vi "handler_file.vi"(8 "error in (no error)":errorcluster, 10 "Server Variables":T1 {"Energy Levels"."E1" format="%_6g"; "Phases"."ExtTriggerDelay" format="%.3g"}, 11 "HTTP Request":T7) -> (0 "error out":errorcluster, 2 "Server Variables 2":T1 {"Energy Levels"."E1" format="%_6g"; "Phases"."ExtTriggerDelay" format="%.3g"}, 3 "HTTP Request out":T7)   [LabVIEW 2011]
uses:
  http_request_response.ctl
  http_request.ctl
  http_field.ctl
  http_response.ctl
  template_field.ctl
  template_field_type.ctl
  Server Variables.ctl
  Phase Parameters.ctl
  Phase Mode.ctl
  Energy Level_.ctl
  Measurement Parameters.ctl
  Results.ctl
  <vilib>/regexp/Match Regular Expression.xnode
panel:
  in  "base path":path=path "c:/nanolyzer/www"
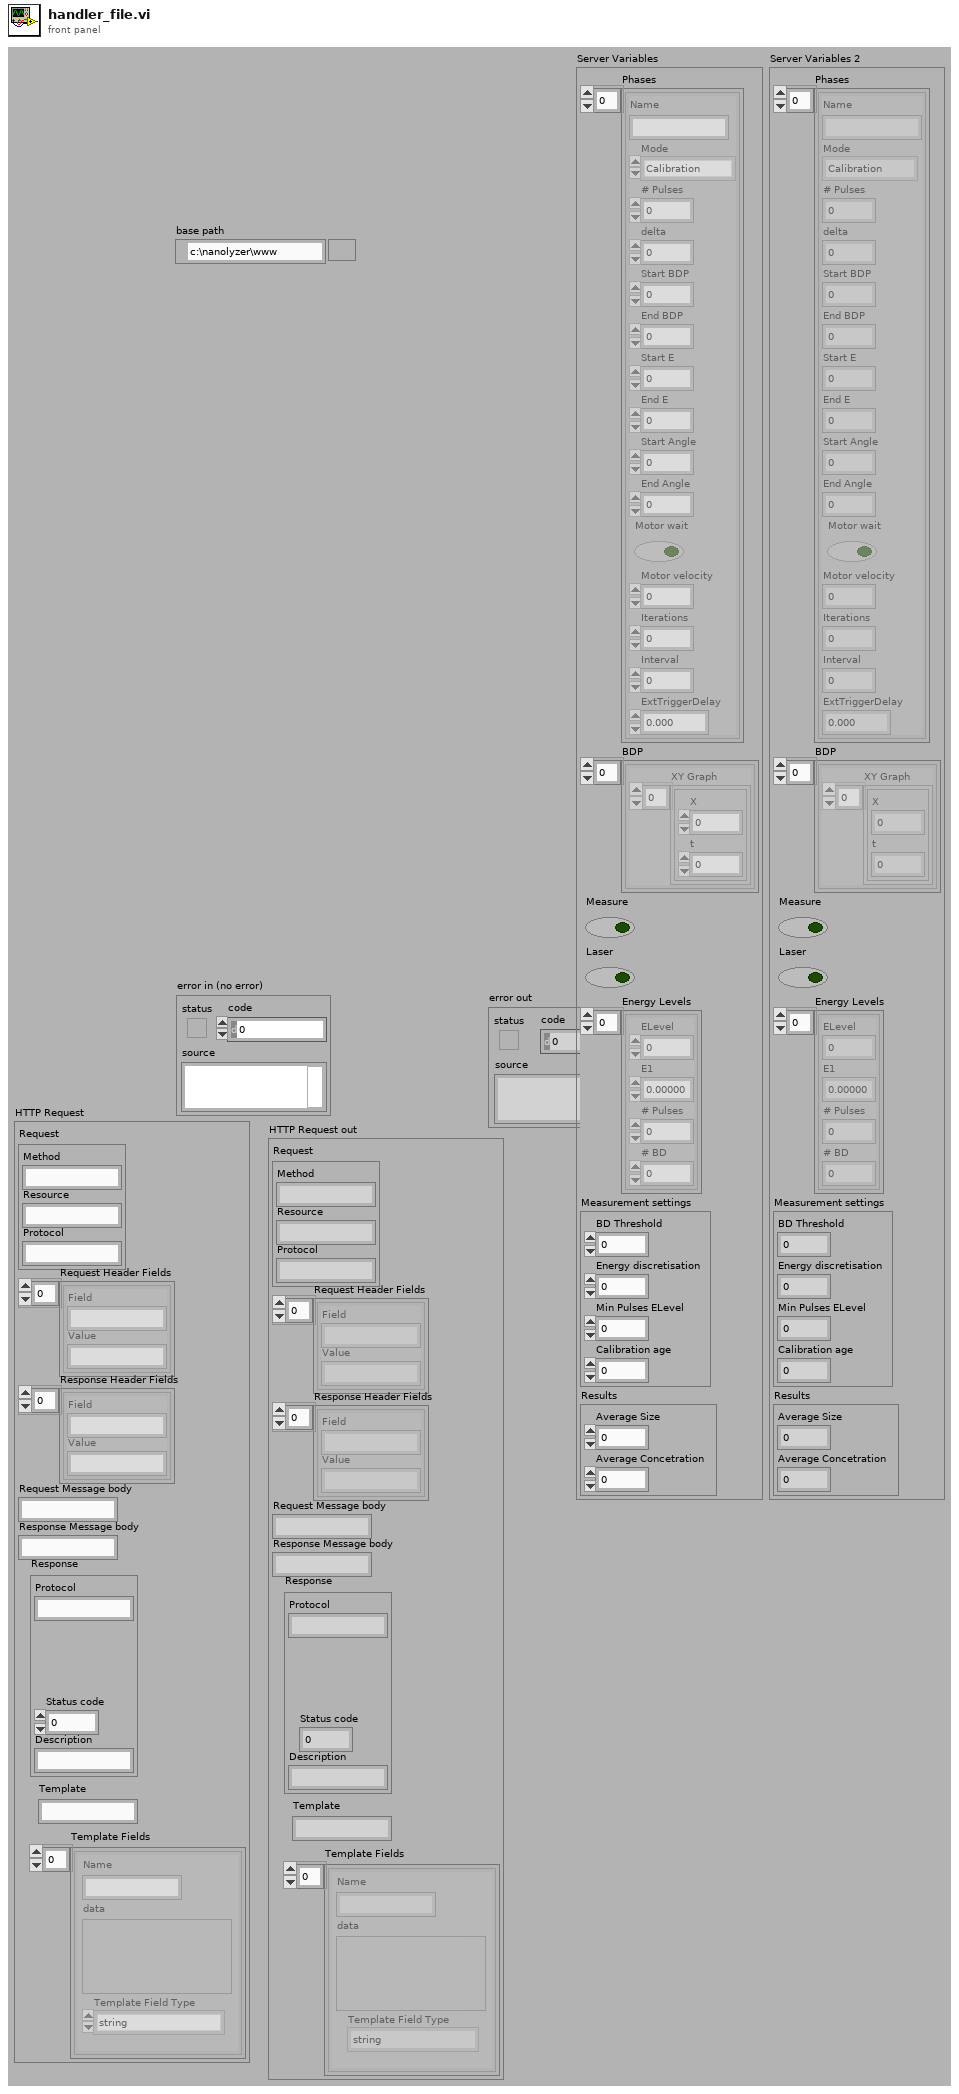
[diagram p1: front panel]
types:
  T1 = typedef "Server Variables.ctl" = cluster{"Phases":T2[], "BDP":cluster{"XY Graph":cluster{"X":dbl, "t":dbl}[]}[], "Measure":bool, "Laser":bool, "Energy Levels":T4[], "Measurement settings":T5, "Results":T6}
  T2 = typedef "Phase Parameters.ctl" = cluster{"Name":string, "Mode":T3, "# Pulses":u32, "delta":dbl, "Start BDP":dbl, "End BDP":dbl, "Start E":dbl, "End E":dbl, "Start Angle":dbl, "End Angle":dbl, "Motor wait":bool, "Motor velocity":dbl, "Iterations":dbl, "Interval":dbl, "ExtTriggerDelay":dbl}
  T3 = typedef "Phase Mode.ctl" = enum16{"Calibration", "Linear", "BDP-Fit", "Raw"}
  T4 = typedef "Energy Level_.ctl" = cluster{"ELevel":dbl, "E1":dbl, "# Pulses":i32, "# BD":i32}
  T5 = typedef "Measurement Parameters.ctl" = cluster{"BD Threshold":dbl, "Energy discretisation":i32, "Min Pulses ELevel":i32, "Calibration age":i32}
  T6 = typedef "Results.ctl" = cluster{"Average Size":dbl, "Average Concetration":dbl}
  T7 = typedef "http_request_response.ctl" = cluster{"Request":T8, "Request Header Fields":T9[], "Response Header Fields":T9[], "Request Message body":string, "Response Message body":string, "Response":T10, "Template":string, "Template Fields":T11[]}
  T8 = typedef "http_request.ctl" = cluster{"Method":string, "Resource":string, "Protocol":string}
  T9 = typedef "http_field.ctl" = cluster{"Field":string, "Value":string}
  T10 = typedef "http_response.ctl" = cluster{"Protocol":string, "Status code":dbl, "Description":string}
  T11 = typedef "template_field.ctl" = cluster{"Name":string, "Template Field Type":T12, "data":variant}
  T12 = typedef "template_field_type.ctl" = enum16{"string", "string array", "number", "number array", "cluster", "cluster array"}
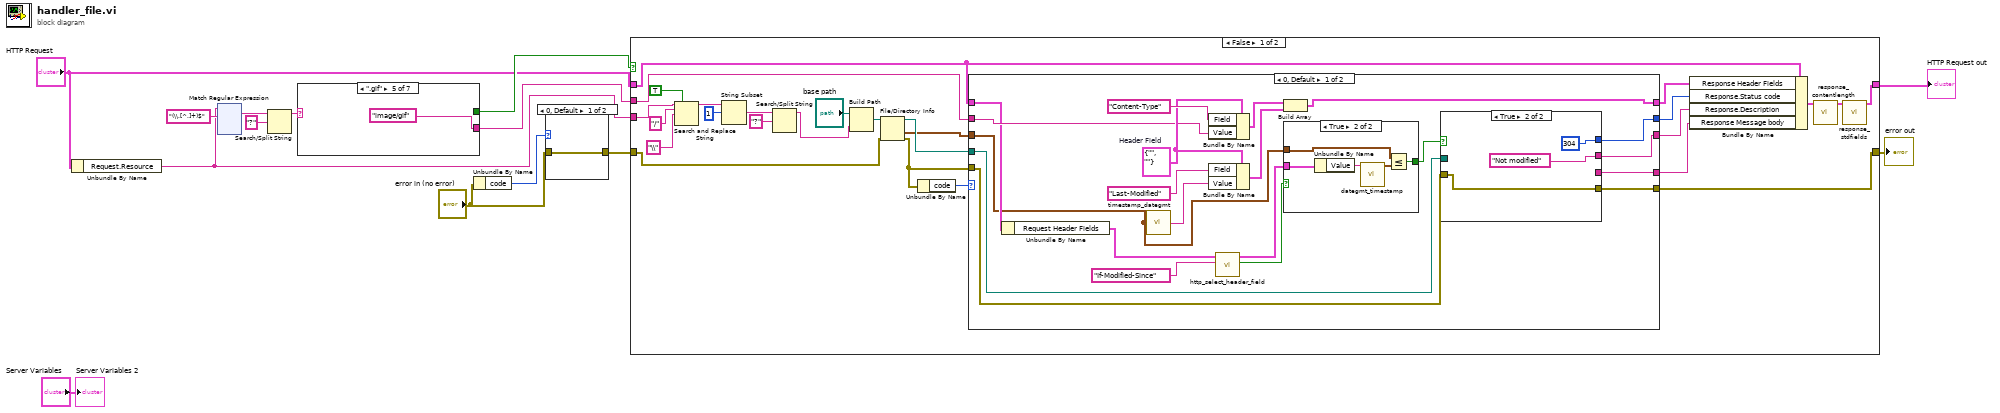
[diagram p0: block diagram]
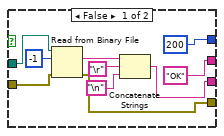
[diagram p2: hidden frame]
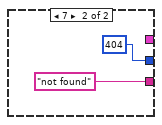
[diagram p4: hidden frame]
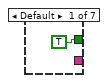
[diagram p6: hidden frame]
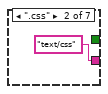
[diagram p7: hidden frame]
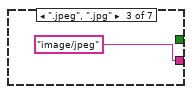
[diagram p8: hidden frame]
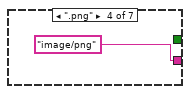
[diagram p9: hidden frame]
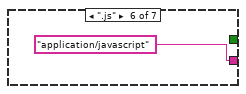
[diagram p10: hidden frame]
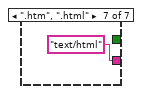
[diagram p11: hidden frame]
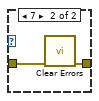
[diagram p12: hidden frame]
diagram:
  n1 = Unbundle By Name("HTTP Request") -> ("Request.Resource"=w5:string)
  n2 = xnode "Match Regular Expression"("input string"=w5, "regular expression"="(\\.[^.]+)$") -> ("whole match"=w2:string)  [unwired: 4 in, 4 out]
  n3 = Search/Split String(string=w2, search string/char (-)="?") -> (substring before match=w1:string)  [unwired: 1 in, 2 out]
  n4 = case shown="\".gif\"" w1 {
    tunnel: [_ "text/css" ("Value") "image/jpeg" ("Value") "image/png" ("Value") "image/gif" ("Value") "application/javascript" ("Value") "text/html" ("Value")] -> w10
    tunnel: [TRUE _ _ _ _ _ _] -> w9
    frame Default {
    }
    frame ".css" {
    }
    frame ".jpeg", ".jpg" {
    }
    frame ".png" {
    }
    frame ".gif" {
    }
    frame ".js" {
    }
    frame ".htm", ".html" {
    }
  }
  n5 = Unbundle By Name("error in (no error)") -> ("code"=w12:i32)
  n6 = case shown="0, Default" w12 {
    tunnel: "error in (no error)" -> [w22 w24]
    tunnel: [w22 w23] -> w6
    frame 0, Default {
    }
    frame 7 {
      n7 = call <vilib>:"Clear Errors.vi"("error in (no error)"=w24) -> ("error out"=w23:errorcluster)  [unwired: 6 in]
    }
  }
  n8 = case shown="False" w9 {
    tunnel: "HTTP Request" -> [w28 w93]
    tunnel: [w47 w92] -> w14
    tunnel: [w42 w93] -> w7
    tunnel: w10 -> [w45 _]
    tunnel: w6 -> [w41 w92]
    tunnel: w5 -> [w33 _]
    frame False {
      n9 = Search and Replace String(replace all?=TRUE ("replace all? (F)"), input string=w33, search string="/", replace string="\\" ("replace string (\"\")")) -> (result string=w37:string)  [unwired: 4 in, 3 out]
      n10 = String Subset(string=w37, offset (0)=1) -> (substring=w26:string)  [unwired: 1 in]
      n11 = Search/Split String(string=w26, search string/char (-)="?") -> (substring before match=w25:string)  [unwired: 1 in, 2 out]
      n12 = Build Path(base path="base path", name or relative path=w25) -> (appended path=w34:path)
      n13 = File/Directory Info(path=w34, error in=w41) -> (path out=w40:path, last mod=w29:timestamp, error out=w39:errorcluster)  [unwired: 4 out]
      n14 = Unbundle By Name(w39) -> ("code"=w38:i32)
      n15 = case shown="0, Default" w38 {
        tunnel: [w71 404] -> w50
        tunnel: [w70 "not found"] -> w49
        tunnel: w40 -> [w69 _]
        tunnel: [w60 _] -> w48
        tunnel: w39 -> [w68 _]
        tunnel: [w67 _] -> w47
        tunnel: [w66 _] -> w46
        tunnel: w29 -> [w52 _]
        tunnel: w45 -> [w58 _]
        tunnel: w28 -> [w53 _]
        frame 0, Default {
          w62 = T9 {"Field"="", "Value"=""}  # Header Field
          n16 = Unbundle By Name(w53) -> ("Request Header Fields"=w54:T9[])
          n17 = call "timestamp_dategmt.vi"("time stamp"=w52) -> ("String"=w61:string)
          n18 = Bundle By Name(cluster=w62, "Field"="Content-Type", "Value"=w58) -> (w59:T9)
          n19 = Bundle By Name(cluster=w62, "Field"="Last-Modified", "Value"=w61) -> (w63:T9)
          n20 = call "http_select_header_field.vi"("Name"="If-Modified-Since", "Request Header Fields"=w54) -> ("found"=w56:bool, "Header Field"=w57:T9)  [unwired: 8 in]
          n21 = Build Array(w59, w63) -> (w66:T9[])
          n22 = case shown="True" w56 {
            tunnel: w57 -> [_ w89]
            tunnel: w52 -> [_ w87]
            tunnel: [_ w85] -> w51
            frame False {
            }
            frame True {
              n23 = Unbundle By Name(w89) -> ("Value"=w88:string)
              n24 = call "dategmt_timestamp.vi"("String"=w88) -> ("time stamp"=w86:timestamp)  [unwired: 10 in]
              n25 = Less Or Equal?(x=w87, y=w86) -> (x <= y?=w85:bool)
            }
          }
          n26 = case shown="True" w51 {
            tunnel: [200 304] -> w71
            tunnel: ["OK" "Not modified"] -> w70
            tunnel: w69 -> [w79 _]
            tunnel: w68 -> [w77 w82]
            tunnel: [w76 w82] -> w67
            tunnel: [w74 _] -> w60
            frame False {
              n27 = Read from Binary File(8:w77, 10:-1 ("count"), 11:w79) -> (0:w76:errorcluster, 2:w75:string)  [unwired: 3 in, 2 out]
              n28 = Concatenate Strings(w75, "\r", "\n") -> (w74:string)
            }
            frame True {
            }
          }
        }
        frame 7 {
        }
      }
      n29 = Bundle By Name(cluster=w28, "Response Header Fields"=w46, "Response.Status code"=w50, "Response.Description"=w49, "Response Message body"=w48) -> (w44:T7)
      n30 = call "response_contentlength.vi"("HTTP Request"=w44) -> ("HTTP Request"=w43:T7)  [unwired: 10 in]
      n31 = call "response_stdfields.vi"("HTTP Request"=w43) -> ("HTTP Request out"=w42:T7)  [unwired: 10 in]
    }
    frame True {
    }
  }
  "error out" <- w14
  "HTTP Request out" <- w7
  "Server Variables 2" <- "Server Variables"
